vi "CRYUpdate Current TS Step.vi"(10 "setup flattened":string, 11 "step index":i32=1) -> ()   [LabVIEW 2013]
uses:
  CRYProject Editor Global.vi
panel:
  in  "Step Name":string
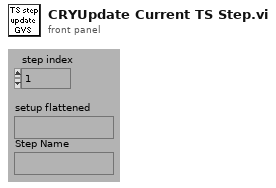
[diagram p1: front panel]
types:
  T1 = typedef "CRYTS.ctl" = cluster{"No.TS":u16, "TS File Path":path, "TS Name":string, "EditStepName":string, "Steps":T2[], "New State":bool, "Change State":bool, "Flattened CurveLib Data":string, "Document Data":string, "EditStepNo":u16, "Operator Start File":string, "Sequence Type":string, "Sequence Language":string}
  T2 = typedef "CRYStep.ctl" = cluster{"No.VI":i32, "Category":string, "StepName":string, "Seq setup flattened":string, "Comment":string, "Steps config.":bool[], "Jump config":i32[], "Start":dbl, "Increment":dbl, "Name":string, "Unit":string, "Y data":u16, "Y prefix":string, "Y dB ref":dbl, "Y unit":string, "Repeat State Array":cluster{"Start":dbl, "Increment":dbl, "Count":i32, "Num":i32}[]}
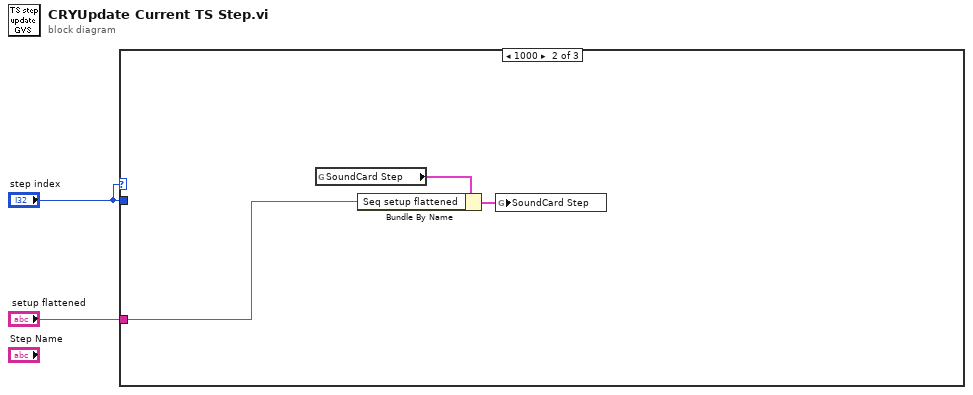
[diagram p0: block diagram]
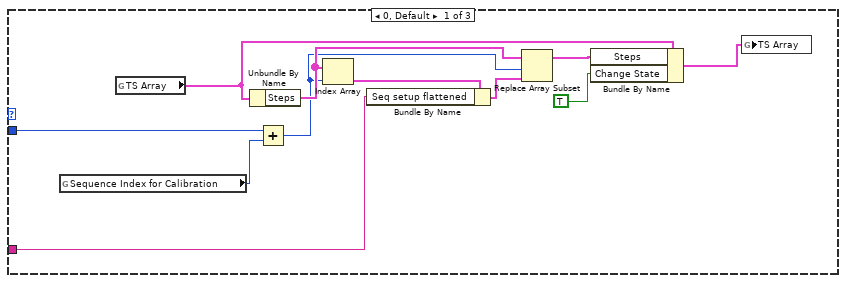
[diagram p2: hidden frame]
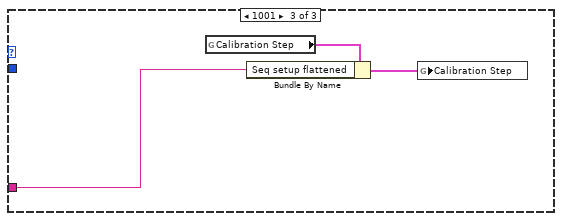
[diagram p3: hidden frame]
diagram:
  n1 = case shown="1000" "step index" {
    tunnel: "setup flattened" -> [w11 w14 w17]
    tunnel: "step index" -> [w5 _ _]
    frame 0, Default {
      n2 = global read "CRYProject Editor Global.vi" "Sequence Index for Calibration"() -> (w3:i32)
      n3 = global read "CRYProject Editor Global.vi" "TS Array"() -> (w7:T1)
      n4 = Unbundle By Name(w7) -> ("Steps"=w9:T2[])
      n5 = Add(x=w5, y=w3) -> (x+y=w4:i32)
      n6 = Index Array(array=w9, index=w4) -> (element=w13:T2)
      n7 = Bundle By Name(cluster=w13, "Seq setup flattened"=w11) -> (w12:T2)
      n8 = Replace Array Subset(array=w9, new element=w12, index=w4) -> (w10:T2[])
      n9 = Bundle By Name(cluster=w7, "Steps"=w10, "Change State"=TRUE ("New State")) -> (w6:T1)
      n10 = global write "CRYProject Editor Global.vi" "TS Array"(w6) -> ()
    }
    frame 1000 {
      n11 = global read "CRYProject Editor Global.vi" "SoundCard Step"() -> (w16:T2)
      n12 = Bundle By Name(cluster=w16, "Seq setup flattened"=w14) -> (w15:T2)
      n13 = global write "CRYProject Editor Global.vi" "SoundCard Step"(w15) -> ()
    }
    frame 1001 {
      n14 = global read "CRYProject Editor Global.vi" "Calibration Step"() -> (w19:T2)
      n15 = Bundle By Name(cluster=w19, "Seq setup flattened"=w17) -> (w18:T2)
      n16 = global write "CRYProject Editor Global.vi" "Calibration Step"(w18) -> ()
    }
  }
